vi "Hilbert Matrix (DBL).vi"(11 "matrix size":i32) -> (0 "error":i32, 3 "Hilbert Matrix":T1)   [LabVIEW 2017, in "NI_AALPro.lvlib"]
uses:
  NI_AALPro.lvlib
  RealMatrix.ctl
  NI_Matrix.lvlib
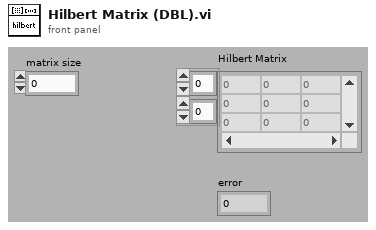
[diagram p1: front panel]
types:
  T1 = typedef "NI_Matrix.lvlib/RealMatrix.ctl" = dbl[][]
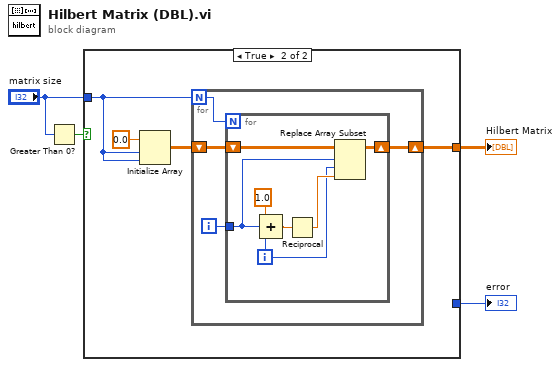
[diagram p0: block diagram]
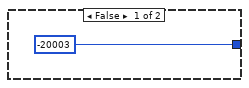
[diagram p2: hidden frame]
diagram:
  n1 = Greater Than 0?(x="matrix size") -> (x > 0?=w3:bool)
  n2 = case shown="True" w3 {
    tunnel: [_ w9] -> w1
    tunnel: [-20003 _] -> w4
    tunnel: "matrix size" -> [_ w7]
    frame False {
    }
    frame True {
      n3 = Initialize Array(0.0 ("element"), w7, w7) -> (w6:dbl[][])
      n4 = for {
        N: w7 -> [w11]
        shift-right: [w10] -> w9
        shift-left: w6 -> [w12]
        i -> [w13]
        n5 = for {
          N: w11 -> [_]
          tunnel: w13 -> [w15]
          shift-right: [w18] -> w10
          shift-left: w12 -> [w17]
          i -> [w14]
          n6 = Compound Arithmetic op=unknown(1.0, w15, w14) -> (w19:dbl)
          n7 = Reciprocal(x=w19) -> (1/x=w16:dbl)
          n8 = Replace Array Subset(array=w17, new element=w16, index (row)=w15, index (col)=w14) -> (w18:dbl[][])
        }
      }
    }
  }
  "Hilbert Matrix" <- w1
  "error" <- w4
